vi "StandTime.vi"(8 "error in (no error)":errorcluster, 11 "time format string":string="%Y-%m-%d %H:%M:%S") -> (0 "error out":errorcluster, 3 "Time":string)   [LabVIEW 2014]
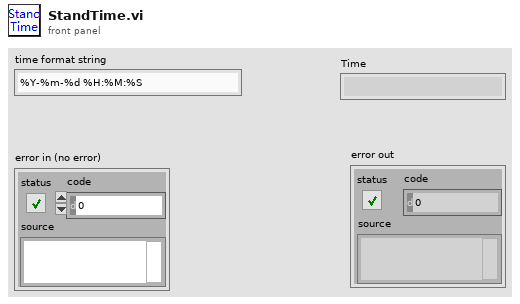
[diagram p1: front panel]
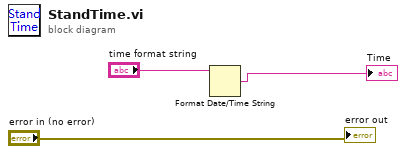
[diagram p0: block diagram]
diagram:
  n1 = Format Date/Time String(time format string (%c)="time format string") -> (date/time string=→"Time":string)  [unwired: 2 in]
  "error out" <- "error in (no error)"
